vi "Result.Numeric Look Up Result Code.vi"(0 "Measurement":T1 {"Status" items=["LOG", "PASS", "FAIL", "ERROR"]}, 1 "error in":errorcluster, 4 "Limits":variant) -> (5 "Measurement Out":T1 {"Status" items=["LOG", "PASS", "FAIL", "ERROR"]})   [LabVIEW 2019]
uses:
  Result.Numeric.ctl
  Result.Limit Type.ctl
  Result.Measurement and Attribute Item Status.ctl
  Result.Test Limit Item.ctl
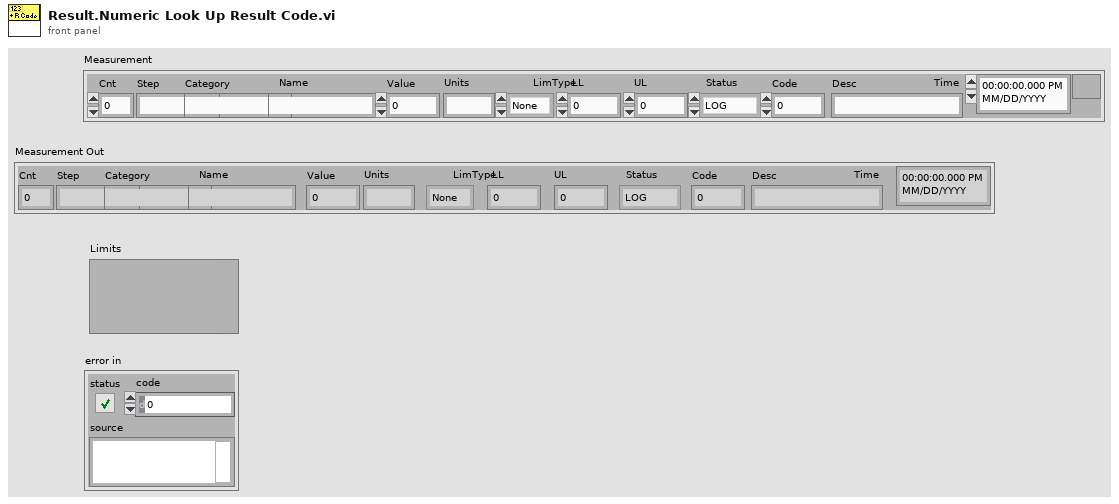
[diagram p1: front panel]
types:
  T1 = typedef "Result.Numeric.ctl" = cluster{"Cnt":i32, "Step":string, "Category":string, "Name":string, "Value":dbl, "Units":string, "LimType":T2, "LL":dbl, "UL":dbl, "Status":T3, "Code":i32, "Desc":string, "Time":timestamp}
  T2 = typedef "Result.Limit Type.ctl" = enum16{"None", "EQ", "NE", "GT", "LT", "GE", "LE", "GTLT", "GELE", "GELT", "GTLE", "LTGT", "LEGE", "LEGT", "LTGE", "Contains", "NotContains"}
  T3 = typedef "Result.Measurement and Attribute Item Status.ctl" = i32
  T4 = typedef "Result.Test Limit Item.ctl" = cluster{"Name":string, "LimType":T2, "LL":string, "UL":string, "Units":string, "FailCode":i32, "FailDesc":string}
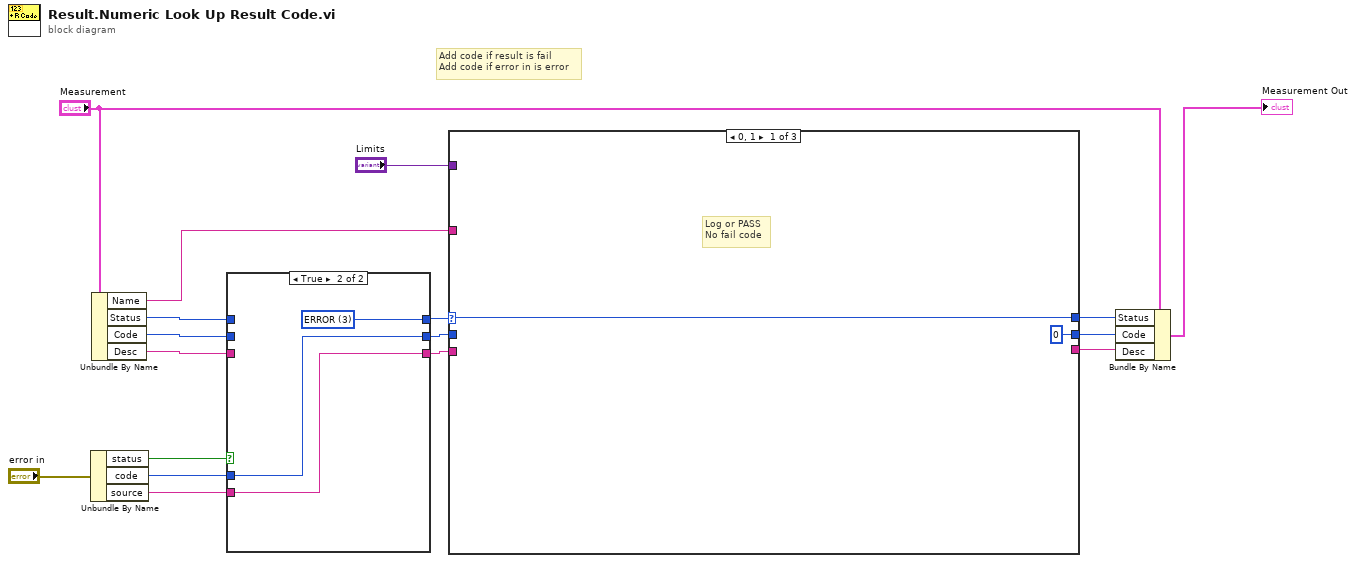
[diagram p0: block diagram]
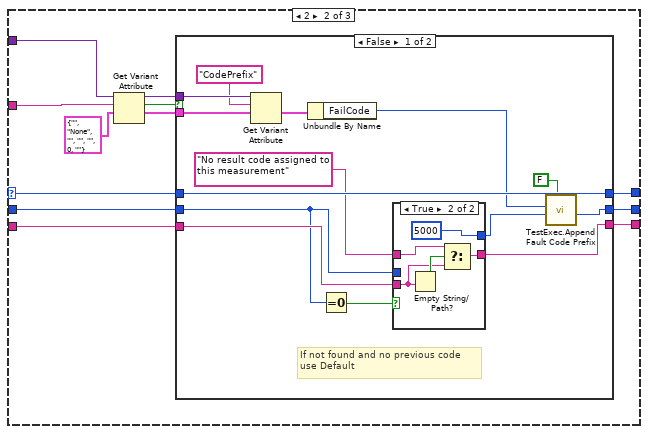
[diagram p2: hidden frame]
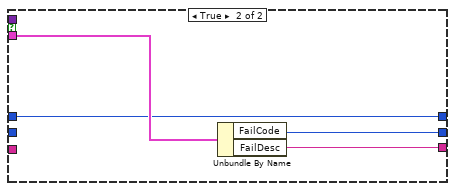
[diagram p4: hidden frame]
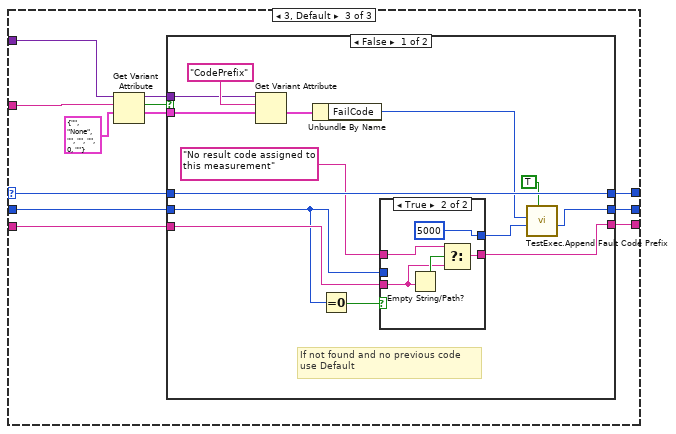
[diagram p5: hidden frame]
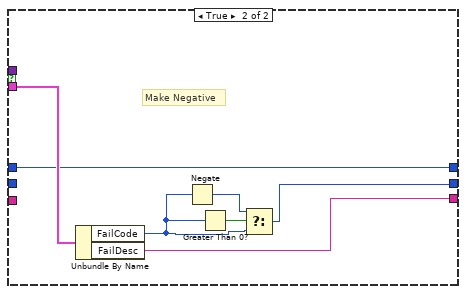
[diagram p7: hidden frame]
diagram:
  # "Add code if result is fail\nAdd code if error in is error"
  n1 = Unbundle By Name("error in") -> ("status"=w14:bool, "code"=w12:i32, "source"=w11:string)
  n2 = Unbundle By Name("Measurement") -> ("Name"=w5:string, "Status"=w13:T3, "Code"=w2:i32, "Desc"=w1:string)
  n3 = case shown="True" w14 {
    tunnel: [w20 w21] -> w10
    tunnel: w13 -> [w20 _]
    tunnel: w12 -> [_ w23]
    tunnel: [w19 w23] -> w8
    tunnel: w11 -> [_ w22]
    tunnel: [w18 w22] -> w7
    tunnel: w2 -> [w19 _]
    tunnel: w1 -> [w18 _]
    frame False {
    }
    frame True {
      w21 = T3 3 items=["LOG", "PASS", "FAIL", "ERROR"] ("Status")
    }
  }
  n4 = case shown="0, 1" w10 {
    selector: w10 -> [w25 w29 w66]
    tunnel: [w25 w28 w65] -> w9
    tunnel: w8 -> [_ w27 w64]
    tunnel: w7 -> [_ w26 w63]
    tunnel: [0 ("FailCode") w32 w69] -> w6
    tunnel: w5 -> [_ w33 w70]
    tunnel: [_ w31 w68] -> w4
    tunnel: "Limits" -> [_ w30 w67]
    frame 0, 1 {
      # "Log or PASS\nNo fail code"
    }
    frame 2 {
      n5 = Get Variant Attribute(Variant=w30, name=w33, default value (empty Variant)=T4 {"Name"="", "LimType"=enum."None", "LL"="", "UL"="", "Units"="", "FailCode"=0, "FailDesc"=""} ("Result.Test Limit Item")) -> (duplicate Variant=w36:variant, found=w37:bool, value=w35:T4)  [unwired: 1 in, 1 out]
      n6 = case shown="False" w37 {
        tunnel: w36 -> [w45 _]
        tunnel: w35 -> [w44 w61]
        tunnel: [w41 w62] -> w32
        tunnel: [w47 w60] -> w31
        tunnel: w29 -> [w51 w59]
        tunnel: [w51 w59] -> w28
        tunnel: w27 -> [w48 _]
        tunnel: w26 -> [w49 _]
        frame False {
          # "If not found and no previous code\nuse Default"
          n7 = Get Variant Attribute(Variant=w45, name="CodePrefix", default value (empty Variant)=w44) -> (value=w42:T4)  [unwired: 1 in, 3 out]
          n8 = Unbundle By Name(w42) -> ("FailCode"=w38:i32)
          n9 = Equal To 0?(x=w48) -> (x = 0?=w50:bool)
          n10 = case shown="True" w50 {
            tunnel: w49 -> [w52 w56]
            tunnel: w48 -> [w53 _]
            tunnel: "No result code assigned to this measurement" ("Desc") -> [_ w55]
            tunnel: [w53 5000 ("Code")] -> w40
            tunnel: [w52 w58] -> w47
            frame False {
            }
            frame True {
              n11 = Empty String/Path?(string/path=w56) -> (empty?=w57:bool)
              n12 = Select(t=w55, s=w57, f=w56) -> (s? t:f=w58:string)
            }
          }
          n13 = call "TestExec.Append Fault Code Prefix.vi"("Positive(F)\\Negative(T)"=FALSE ("Negative(TY)/Positive(F)"), "FaultCode"=w40, "FaultCode Prefix"=w38) -> ("New Fault Code"=w41:i32)  [unwired: 8 in]
        }
        frame True {
          n14 = Unbundle By Name(w61) -> ("FailCode"=w62:i32, "FailDesc"=w60:string)
        }
      }
    }
    frame 3, Default {
      n15 = Get Variant Attribute(Variant=w67, name=w70, default value (empty Variant)=T4 {"Name"="", "LimType"=enum."None", "LL"="", "UL"="", "Units"="", "FailCode"=0, "FailDesc"=""} ("Result.Test Limit Item")) -> (duplicate Variant=w73:variant, found=w74:bool, value=w72:T4)  [unwired: 1 in, 1 out]
      n16 = case shown="False" w74 {
        tunnel: w73 -> [w80 _]
        tunnel: w72 -> [w79 w102]
        tunnel: [w78 w98] -> w69
        tunnel: [w84 w101] -> w68
        tunnel: w66 -> [w88 w100]
        tunnel: [w88 w100] -> w65
        tunnel: w64 -> [w85 _]
        tunnel: w63 -> [w86 _]
        frame False {
          # "If not found and no previous code\nuse Default"
          n17 = Get Variant Attribute(Variant=w80, name="CodePrefix", default value (empty Variant)=w79) -> (value=w81:T4)  [unwired: 1 in, 3 out]
          n18 = Unbundle By Name(w81) -> ("FailCode"=w75:i32)
          n19 = Equal To 0?(x=w85) -> (x = 0?=w87:bool)
          n20 = case shown="True" w87 {
            tunnel: w86 -> [w89 w93]
            tunnel: w85 -> [w90 _]
            tunnel: "No result code assigned to this measurement" ("Desc") -> [_ w92]
            tunnel: [w90 5000 ("Code")] -> w77
            tunnel: [w89 w95] -> w84
            frame False {
            }
            frame True {
              n21 = Empty String/Path?(string/path=w93) -> (empty?=w94:bool)
              n22 = Select(t=w92, s=w94, f=w93) -> (s? t:f=w95:string)
            }
          }
          n23 = call "TestExec.Append Fault Code Prefix.vi"("Positive(F)\\Negative(T)"=TRUE ("Positive(F)\\Negative(T)"), "FaultCode"=w77, "FaultCode Prefix"=w75) -> ("New Fault Code"=w78:i32)  [unwired: 8 in]
        }
        frame True {
          # "Make Negative"
          n24 = Unbundle By Name(w102) -> ("FailCode"=w96:i32, "FailDesc"=w101:string)
          n25 = Negate(x=w96) -> (-x=w97:i32)
          n26 = Greater Than 0?(x=w96) -> (x > 0?=w99:bool)
          n27 = Select(t=w97, s=w99, f=w96) -> (s? t:f=w98:i32)
        }
      }
    }
  }
  n28 = Bundle By Name(cluster="Measurement", "Status"=w9, "Code"=w6, "Desc"=w4) -> (→"Measurement Out":T1)
